vi "FolloWinDemo.vi"() -> ()   [LabVIEW 2023]
doc: "TOP VI of this project that demonstrates the use of \"FolloWin\" class. \n\nRun this VI to run the demo"
uses:
  FolloWin Class/FolloWin.lvclass
panel:
  in  "Intensity Graph":dbl[][](graph)
  in  "XY Graph":cluster{"X":dbl, "Y":dbl}[](graph)
  in  "Transparency":u8=30 max=100 step=1
  in  "Update\ndelay(ms)":u32=15 max=100000
  in  "Y offset":i32=30 min=-10000 max=10000
  in  "X offset":i32=30 min=-10000 max=10000
  in  "Width":u32=130 max=100000
  in  "Height":u32=50 max=100000
  # "FolloWin Demonstration VI"
  # "Description\n\nThis is a demonstration of the \"FolloWin\" Class. \nit's an object that implements an information window that follows the mouse cursor.\n\n\nTo use\n\nRun this VI and move the mouse  cursor over the \ngraphs.\n\nPress the mouse button to switch between position and line/measuring modes. \n\nTo stop the demonstration  use the X button on the top right."
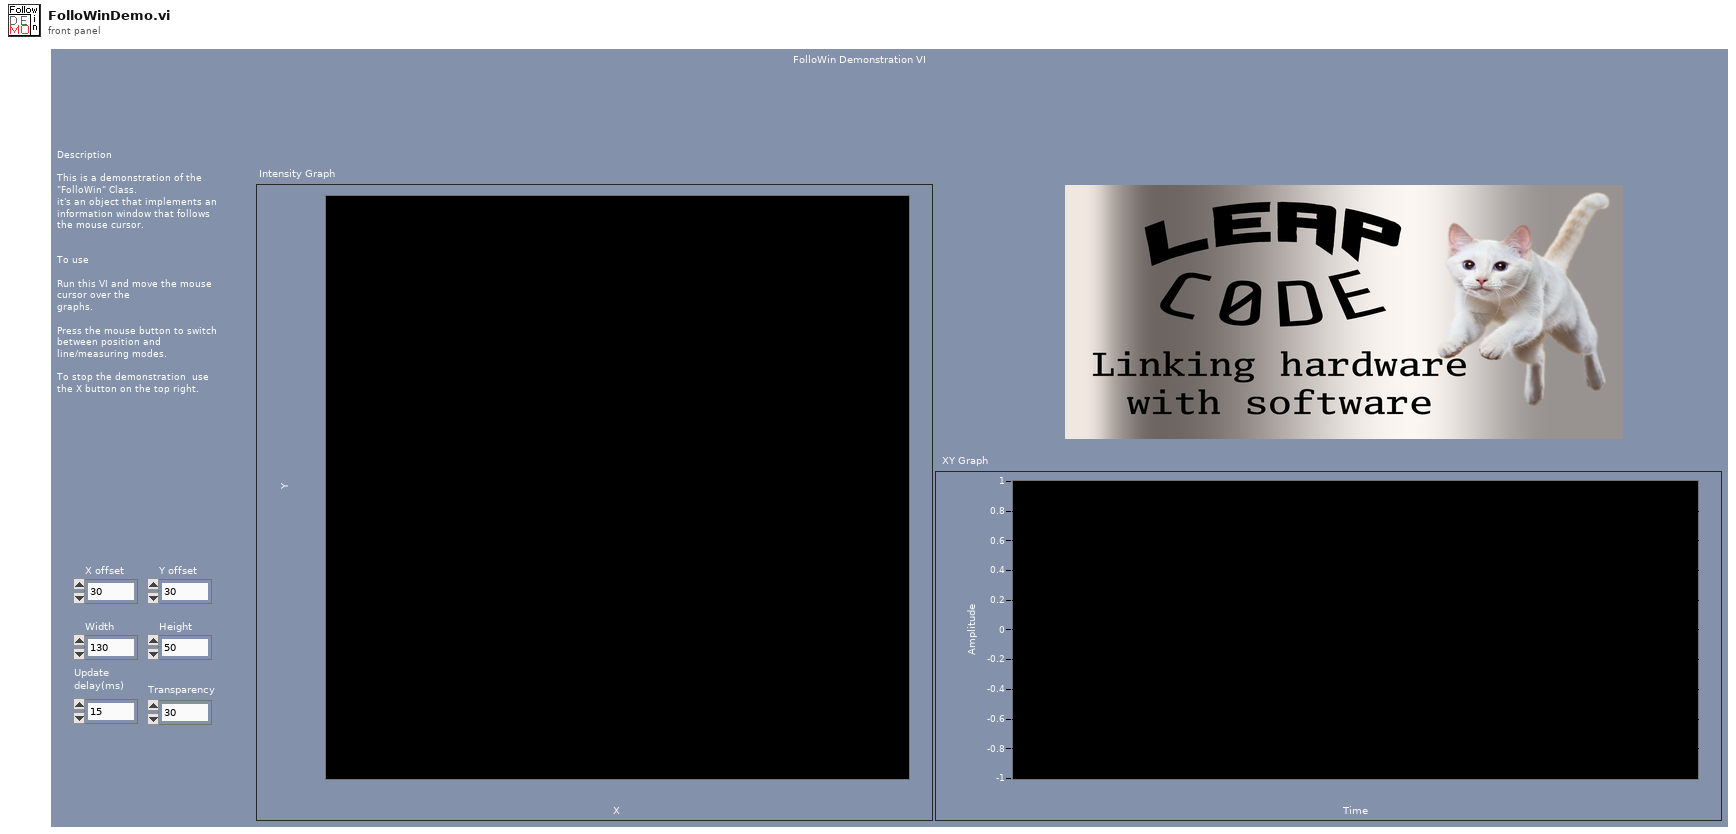
[diagram p1: front panel]
types:
  T1 = typedef "LVRectTypeDef.ctl" = cluster{"Left":i16, "Top":i16, "Right":i16, "Bottom":i16}
  T2 = typedef "LVPoint32TypeDef.ctl" = cluster{"Horizontal":i32, "Vertical":i32}
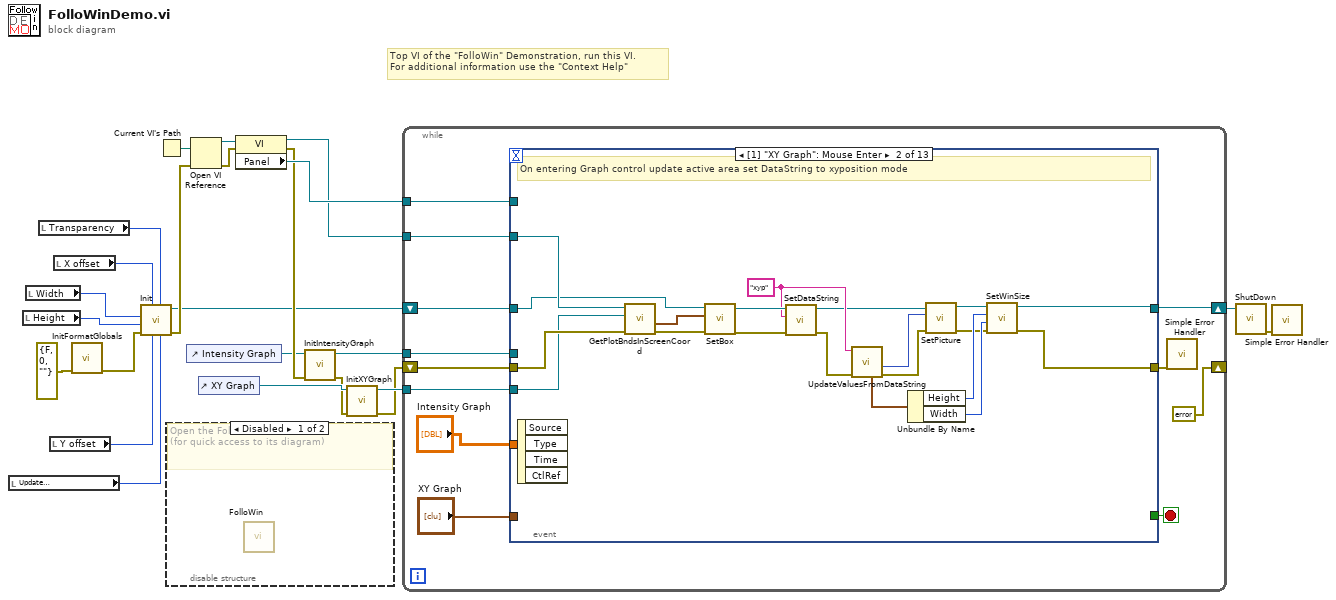
[diagram p0: block diagram]
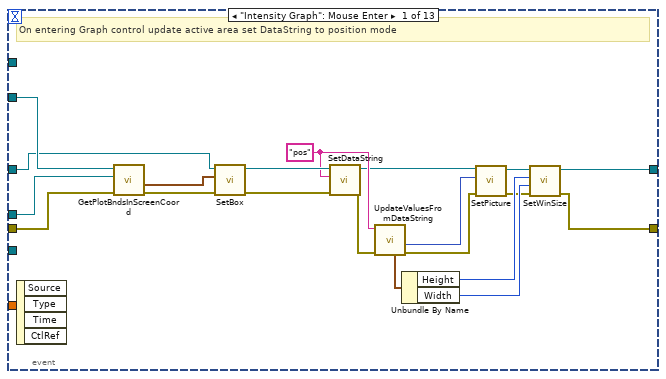
[diagram p3: hidden frame]
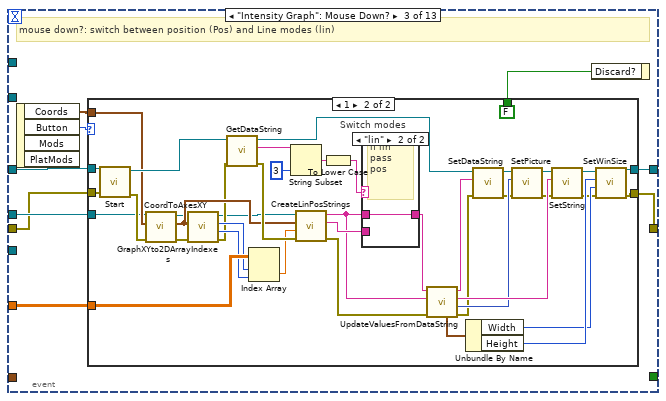
[diagram p4: hidden frame]
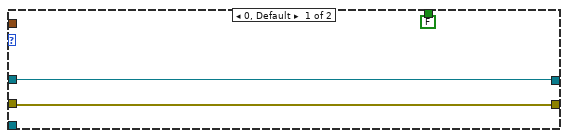
[diagram p5: hidden frame]
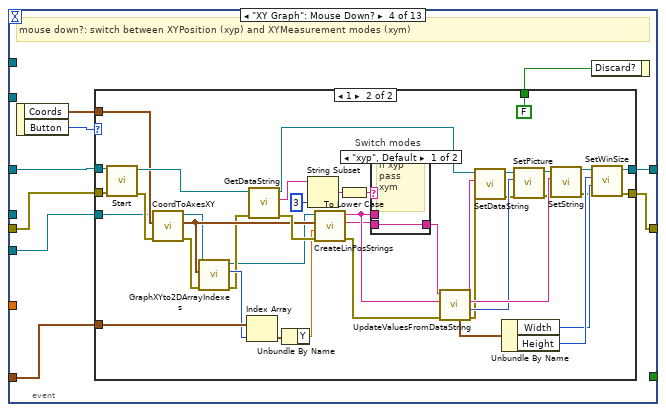
[diagram p7: hidden frame]
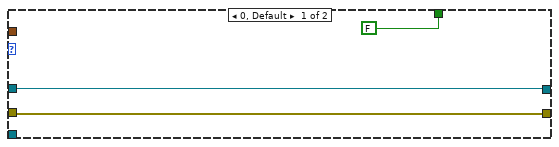
[diagram p8: hidden frame]
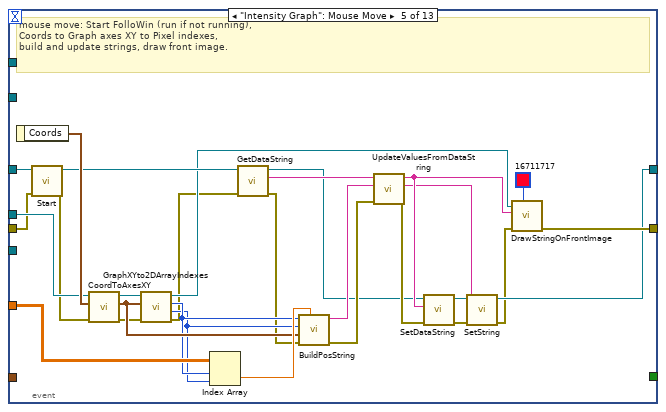
[diagram p10: hidden frame]
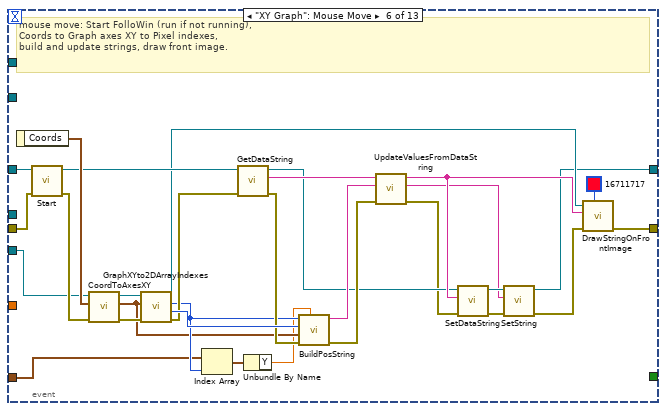
[diagram p11: hidden frame]
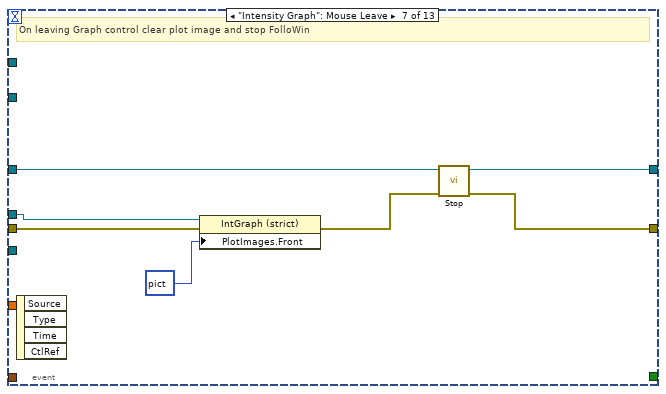
[diagram p12: hidden frame]
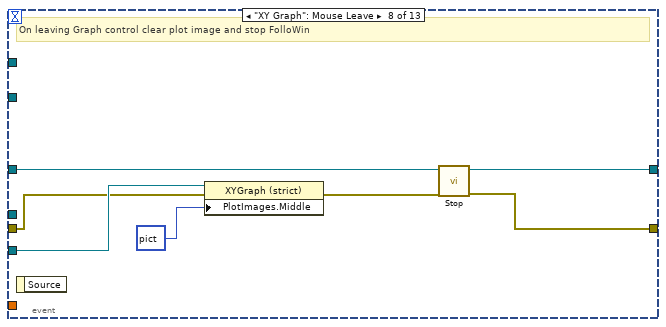
[diagram p13: hidden frame]
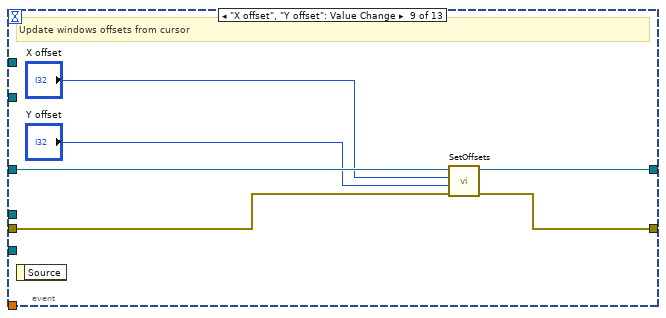
[diagram p14: hidden frame]
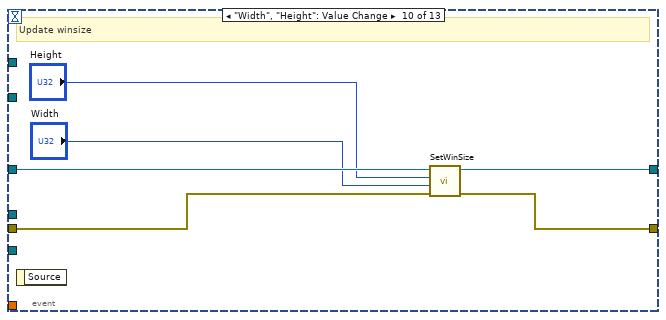
[diagram p15: hidden frame]
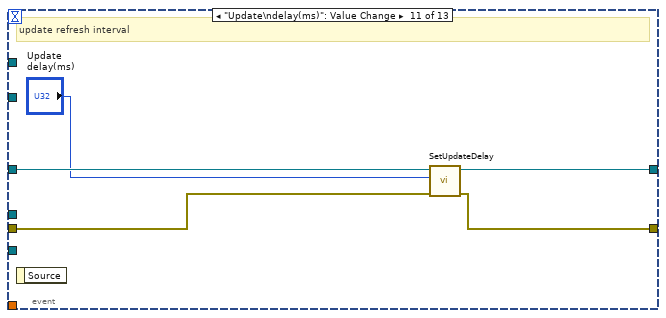
[diagram p16: hidden frame]
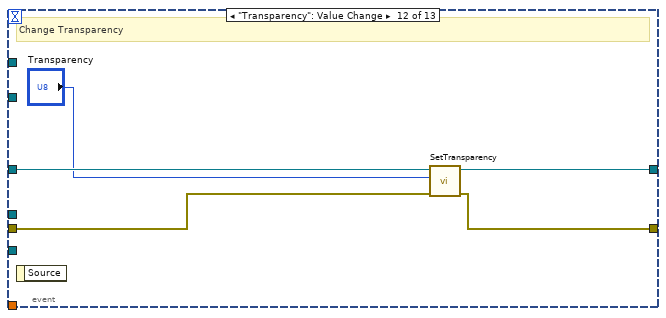
[diagram p17: hidden frame]
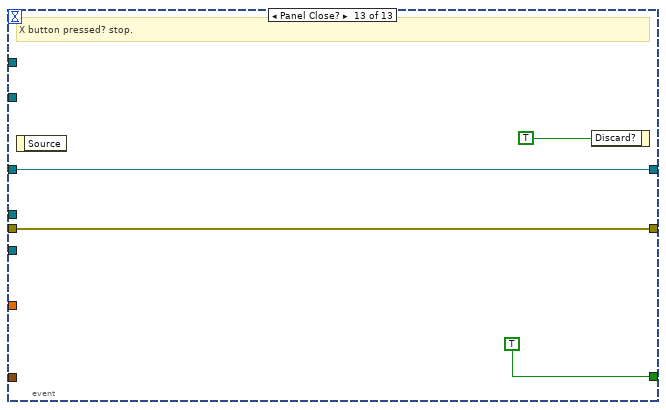
[diagram p18: hidden frame]
diagram:
  # "Top VI of the \"FolloWin\" Demonstration, run this VI. \nFor additional information use the \"Context Help\""
  n1 = local read "Update\ndelay(ms)"() -> (w12:u32)
  n2 = local read "Height"() -> (w23:u32)
  n3 = local read "Width"() -> (w24:u32)
  n4 = local read "Transparency"() -> (w11:u8)
  n5 = local read "Y offset"() -> (w17:i32)
  n6 = local read "X offset"() -> (w18:i32)
  n7 = call "InitFormatGlobals.vi"("error in (no error)"=errorcluster {"status"=FALSE, "code"=0, "source"=""}) -> ("error out"=w6:errorcluster)  [unwired: 10 in]
  n8 = call "Init.vi"("Update delay (ms)"=w12, "Transparency"=w11, "Y offset"=w17, "X offset"=w18, "error in (no error)"=w6, "WinHeight"=w23, "WinWidth"=w24) -> ("error out"=w15:errorcluster, "FolloWin out"=w10:refnum<class "FolloWin.lvclass">)  [unwired: 3 in]
  n9 = Current VI's Path() -> (path=w21:path)
  n10 = disable-structure "Diagram Disable Structure" shown="Disabled" {
    frame Disabled {
      # "Open the FolloWin GUI window\n(for quick access to its diagram)"
      n11 = call "FolloWin.vi"() -> ()  [unwired: 12 in]
    }
    frame Enabled {
    }
  }
  n12 = control-ref of="Intensity Graph"() -> (w1:refnum<vi>)
  n13 = Open VI Reference(vi path=w21, error in (no error)=w15) -> (vi reference=w20:refnum<vi>, error out=w16:errorcluster)  [unwired: 4 in]
  n14 = control-ref of="XY Graph"() -> (w5:refnum<vi>)
  n15 = property on="Property Node" class="VI"(reference=w20, error in=w16) -> (reference out=w13:refnum<vi>, error out=w14:errorcluster, "Panel"=w19:refnum<vi>)
  n16 = call "InitIntensityGraph.vi"("error in (no error)"=w14, "IntensityGraph in"=w1) -> ("error out"=w2:errorcluster, "IntensityGraph out"=w22:refnum<vi>)  [unwired: 8 in]
  n17 = call "InitXYGraph.vi"("error in (no error)"=w2, "XYGraph in"=w5) -> ("error out"=w3:errorcluster, "XYGraph out"=w4:refnum<vi>)  [unwired: 8 in]
  n18 = while {
    shift-right: [w35] -> w9
    shift-left: w10 -> [w36]
    shift-right: [errorcluster {"status"=FALSE, "code"=0, "source"=""} ("error out")] -> _
    shift-left: w3 -> [w34]
    tunnel: w22 -> [w32]
    tunnel: w19 -> [w31]
    tunnel: w13 -> [w30]
    tunnel: w4 -> [w27]
    stop <- w29 stop-if-true
    n19 = event shown="[1] \"XY Graph\": Mouse Enter" {
      selector: _ -> [_ _ _ _ _ _ _ _ _ _ _ _ _]
      dyn-events: _ -> [_ _ _ _ _ _ _ _ _ _ _ _ _]
      timeout: _ -> [_ _ _ _ _ _ _ _ _ _ _ _ _]
      tunnel: w36 -> [w52 w73 w85 w140 w211 w244 w250 w257 w265 w271 w276 w281 w282]
      tunnel: [w37 w66 w84 w139 w190 w218 w252 w259 w264 w266 w273 w278 w282] -> w35
      tunnel: w34 -> [w51 w72 w80 w137 w198 w233 w249 w255 w262 w268 w275 w280 w283]
      tunnel: [w46 w62 w77 w136 w191 w226 w251 w258 w263 w267 w274 w279 w283] -> w33
      tunnel: "Intensity Graph" -> [_ _ w81 _ w214 _ _ _ _ _ _ _ _]
      tunnel: w32 -> [w54 _ w82 _ w205 _ w247 _ _ _ _ _ _]
      tunnel: w31 -> [_ _ _ _ _ _ _ _ _ _ _ _ _]
      tunnel: w30 -> [w55 w75 _ _ _ _ _ _ _ _ _ _ _]
      tunnel: [_ _ _ _ _ _ _ _ _ _ _ _ TRUE] -> w29
      tunnel: w27 -> [_ w69 _ w133 _ w224 _ w256 _ _ _ _ _]
      tunnel: "XY Graph" -> [_ _ _ w132 _ w220 _ _ _ _ _ _ _]
      event "Intensity Graph": Mouse Enter {
        w48 = "pos" ("DataString")
        # "On entering Graph control update active area set DataString to position mode"
        n20 = event-data() -> ()  [unwired: 1 in, 4 out]
        n21 = call "GetPlotBndsInScreenCoord.vi"("error in (no error)"=w51, "IntensityGraph in"=w54, "VI in"=w55) -> ("error out"=w53:errorcluster, "Bounds Screen Coordinates"=w56:T1)  [unwired: 6 in, 1 out]
        n22 = call "SetBox.vi"("error in (no error)"=w53, "Box"=w56, "FolloWin in"=w52) -> ("error out"=w49:errorcluster, "FolloWin out"=w50:refnum<class "FolloWin.lvclass">)  [unwired: 7 in]
        n23 = call-dynamic "SetDataString.vi"("error in (no error)"=w49, "DataString"=w48, "FolloWin in"=w50) -> ("error out"=w47:errorcluster, "FolloWin out"=w41:refnum<class "FolloWin.lvclass">)  [unwired: 7 in]
        n24 = call "UpdateValuesFromDataString.vi"("error In"=w47, "Current String"=w48) -> ("error out"=w39:errorcluster, "BG Image"=w42:picture, "WinSize"=w45:cluster{"Width":i32, "Height":i32})  [unwired: 5 in, 2 out]
        n25 = Unbundle By Name(w45) -> ("Height"=w43:i32, "Width"=w44:i32)
        n26 = call-dynamic "SetPicture.vi"("error in (no error)"=w39, "Picture"=w42, "FolloWin in"=w41) -> ("error out"=w38:errorcluster, "FolloWin out"=w40:refnum<class "FolloWin.lvclass">)  [unwired: 7 in]
        n27 = call-dynamic "SetWinSize.vi"("error in (no error)"=w38, "Width"=w44, "Height"=w43, "FolloWin in"=w40) -> ("error out"=w46:errorcluster, "FolloWin out"=w37:refnum<class "FolloWin.lvclass">)  [unwired: 6 in]
      }
      event "XY Graph": Mouse Enter {
        w68 = "xyp" ("DataString")
        # "On entering Graph control update active area set DataString to xyposition mode"
        n28 = event-data() -> ()  [unwired: 1 in, 4 out]
        n29 = call "GetPlotBndsInScreenCoord.vi"("error in (no error)"=w72, "IntensityGraph in"=w69, "VI in"=w75) -> ("error out"=w74:errorcluster, "Bounds Screen Coordinates"=w76:T1)  [unwired: 6 in, 1 out]
        n30 = call "SetBox.vi"("error in (no error)"=w74, "Box"=w76, "FolloWin in"=w73) -> ("error out"=w70:errorcluster, "FolloWin out"=w71:refnum<class "FolloWin.lvclass">)  [unwired: 7 in]
        n31 = call-dynamic "SetDataString.vi"("error in (no error)"=w70, "DataString"=w68, "FolloWin in"=w71) -> ("error out"=w67:errorcluster, "FolloWin out"=w61:refnum<class "FolloWin.lvclass">)  [unwired: 7 in]
        n32 = call "UpdateValuesFromDataString.vi"("error In"=w67, "Current String"=w68) -> ("error out"=w58:errorcluster, "BG Image"=w59:picture, "WinSize"=w65:cluster{"Width":i32, "Height":i32})  [unwired: 5 in, 2 out]
        n33 = Unbundle By Name(w65) -> ("Height"=w63:i32, "Width"=w64:i32)
        n34 = call-dynamic "SetPicture.vi"("error in (no error)"=w58, "Picture"=w59, "FolloWin in"=w61) -> ("error out"=w57:errorcluster, "FolloWin out"=w60:refnum<class "FolloWin.lvclass">)  [unwired: 7 in]
        n35 = call-dynamic "SetWinSize.vi"("error in (no error)"=w57, "Width"=w64, "Height"=w63, "FolloWin in"=w60) -> ("error out"=w62:errorcluster, "FolloWin out"=w66:refnum<class "FolloWin.lvclass">)  [unwired: 6 in]
      }
      event "Intensity Graph": Mouse Down? {
        # "mouse down?: switch between position (Pos) and Line modes (lin)"
        n36 = event-data() -> ("Coords"=w83:T2, "Button"=w79:u16)  [unwired: 1 in, 2 out]
        n37 = case shown="1" w79 {
          tunnel: w85 -> [w88 w127]
          tunnel: [w88 w92] -> w84
          tunnel: w83 -> [_ w125]
          tunnel: w82 -> [_ w110]
          tunnel: w81 -> [_ w115]
          tunnel: w80 -> [w86 w119]
          tunnel: [FALSE ("Discard?") FALSE ("Discard?")] -> w78
          tunnel: [w86 w93] -> w77
          frame 0, Default {
          }
          frame 1 {
            n38 = call "Start.vi"("error in (no error)"=w119, "FolloWin in"=w127) -> ("error out"=w118:errorcluster, "FolloWin out"=w129:refnum<class "FolloWin.lvclass">)  [unwired: 8 in]
            n39 = call "CoordToAxesXY.vi"("error in (no error)"=w118, "Coords"=w125, "IntensityGraph in"=w110) -> ("error out"=w109:errorcluster, "XY"=w113:cluster{"X":dbl, "Y":dbl}, "IntensityGraph out"=w107:refnum<vi>)  [unwired: 6 in]
            n40 = call "GraphXYto2DArrayIndexes.vi"("error in (no error)"=w109, "XY"=w113, "IntensityGraph in"=w107) -> ("error out"=w108:errorcluster, "Y Index"=w111:i32, "X Index"=w112:i32, "reference out"=w106:refnum<vi>)  [unwired: 5 in]
            n41 = call-dynamic "GetDataString.vi"("error in (no error)"=w108, "FolloWin in"=w129) -> ("error out"=w126:errorcluster, "DataString"=w123:string, "FolloWin out"=w97:refnum<class "FolloWin.lvclass">)  [unwired: 7 in]
            n42 = Index Array(array=w115, index (row)=w112, index (col)=w111) -> (element=w114:dbl)
            n43 = String Subset(string=w123, length (rest)=3 ("length (rest)")) -> (substring=w104:string)  [unwired: 1 in]
            n44 = call "CreateLinPosStrings.vi"("error in (no error)"=w126, "Z/F(x) val"=w114, "Coord"=w113, "IntensityGraph in"=w106) -> ("error out"=w117:errorcluster, "Lin String out"=w121:string, "Pos String out"=w105:string)  [unwired: 5 in]
            n45 = To Lower Case(string=w104) -> (all lower case string=w103:string)
            n46 = case "Switch modes" shown="\"lin\"" w103 {
              tunnel: w121 -> [w130 _]
              tunnel: [w130 w131] -> w120
              tunnel: w105 -> [_ w131]
              frame "pos", Default {
                # "if pos\npass lin"
              }
              frame "lin" {
                # "if lin \npass pos"
              }
            }
            n47 = call "UpdateValuesFromDataString.vi"("error In"=w117, "New point string"=w105, "Current String"=w120) -> ("error out"=w95:errorcluster, "BG Image"=w101:picture, "DisplayString"=w124:string, "DataString"=w128:string, "WinSize"=w100:cluster{"Width":i32, "Height":i32})  [unwired: 4 in]
            n48 = Unbundle By Name(w100) -> ("Width"=w98:i32, "Height"=w99:i32)
            n49 = call-dynamic "SetDataString.vi"("error in (no error)"=w95, "DataString"=w128, "FolloWin in"=w97) -> ("error out"=w96:errorcluster, "FolloWin out"=w89:refnum<class "FolloWin.lvclass">)  [unwired: 7 in]
            n50 = call-dynamic "SetPicture.vi"("error in (no error)"=w96, "Picture"=w101, "FolloWin in"=w89) -> ("error out"=w102:errorcluster, "FolloWin out"=w90:refnum<class "FolloWin.lvclass">)  [unwired: 7 in]
            n51 = call-dynamic "SetString.vi"("error in (no error)"=w102, "String Text"=w124, "FolloWin in"=w90) -> ("error out"=w94:errorcluster, "FolloWin out"=w91:refnum<class "FolloWin.lvclass">)  [unwired: 7 in]
            n52 = call-dynamic "SetWinSize.vi"("error in (no error)"=w94, "Width"=w98, "Height"=w99, "FolloWin in"=w91) -> ("error out"=w93:errorcluster, "FolloWin out"=w92:refnum<class "FolloWin.lvclass">)  [unwired: 6 in]
          }
        }
        n53 = event-data ("Event Filter Node")("Discard?"=w78) -> ()  [unwired: 1 in, 1 out]
      }
      event "XY Graph": Mouse Down? {
        # "mouse down?: switch between XYPosition (xyp) and XYMeasurement modes (xym)"
        n54 = event-data() -> ("Coords"=w138:T2, "Button"=w135:u16)  [unwired: 1 in]
        n55 = case shown="1" w135 {
          tunnel: w140 -> [w143 w182]
          tunnel: [w143 w154] -> w139
          tunnel: w138 -> [_ w180]
          tunnel: w133 -> [_ w168]
          tunnel: w137 -> [w142 w176]
          tunnel: [w142 w155] -> w136
          tunnel: [FALSE ("Discard?") FALSE ("Discard?")] -> w134
          tunnel: w132 -> [_ w172]
          frame 0, Default {
          }
          frame 1 {
            n56 = call "Start.vi"("error in (no error)"=w176, "FolloWin in"=w182) -> ("error out"=w175:errorcluster, "FolloWin out"=w184:refnum<class "FolloWin.lvclass">)  [unwired: 8 in]
            n57 = call "CoordToAxesXY.vi"("error in (no error)"=w175, "Coords"=w180, "IntensityGraph in"=w168) -> ("error out"=w166:errorcluster, "XY"=w169:cluster{"X":dbl, "Y":dbl}, "IntensityGraph out"=w164:refnum<vi>)  [unwired: 6 in]
            n58 = call "GraphXYto2DArrayIndexes.vi"("error in (no error)"=w166, "XY"=w169, "IntensityGraph in"=w164) -> ("error out"=w165:errorcluster, "X Index"=w167:i32, "reference out"=w163:refnum<vi>)  [unwired: 5 in, 1 out]
            n59 = Index Array(array=w172, index=w167) -> (element=w171:cluster{"X":dbl, "Y":dbl})
            n60 = call-dynamic "GetDataString.vi"("error in (no error)"=w165, "FolloWin in"=w184) -> ("error out"=w181:errorcluster, "DataString"=w178:string, "FolloWin out"=w149:refnum<class "FolloWin.lvclass">)  [unwired: 7 in]
            n61 = Unbundle By Name(w171) -> ("Y"=w170:dbl)
            n62 = String Subset(string=w178, length (rest)=3 ("length (rest)")) -> (substring=w162:string)  [unwired: 1 in]
            n63 = call "CreateLinPosStrings.vi"("error in (no error)"=w181, "Z/F(x) val"=w170, "Coord"=w169, "IntensityGraph in"=w163) -> ("error out"=w174:errorcluster, "Lin String out"=w145:string, "Pos String out"=w146:string)  [unwired: 5 in]
            n64 = To Lower Case(string=w162) -> (all lower case string=w147:string)
            n65 = case "Switch modes" shown="\"xyp\", Default" w147 {
              tunnel: w145 -> [w185 _]
              tunnel: [w185 w186] -> w144
              tunnel: w146 -> [_ w186]
              frame "xyp", Default {
                # "if xyp pass xym"
              }
              frame "xym" {
                # "if xym \npass xyp"
              }
            }
            n66 = call "UpdateValuesFromDataString.vi"("error In"=w174, "New point string"=w146, "Current String"=w144) -> ("error out"=w148:errorcluster, "BG Image"=w160:picture, "DisplayString"=w179:string, "DataString"=w183:string, "WinSize"=w156:cluster{"Width":i32, "Height":i32})  [unwired: 4 in]
            n67 = call-dynamic "SetDataString.vi"("error in (no error)"=w148, "DataString"=w183, "FolloWin in"=w149) -> ("error out"=w151:errorcluster, "FolloWin out"=w150:refnum<class "FolloWin.lvclass">)  [unwired: 7 in]
            n68 = Unbundle By Name(w156) -> ("Width"=w157:i32, "Height"=w158:i32)
            n69 = call-dynamic "SetPicture.vi"("error in (no error)"=w151, "Picture"=w160, "FolloWin in"=w150) -> ("error out"=w159:errorcluster, "FolloWin out"=w161:refnum<class "FolloWin.lvclass">)  [unwired: 7 in]
            n70 = call-dynamic "SetString.vi"("error in (no error)"=w159, "String Text"=w179, "FolloWin in"=w161) -> ("error out"=w152:errorcluster, "FolloWin out"=w153:refnum<class "FolloWin.lvclass">)  [unwired: 7 in]
            n71 = call-dynamic "SetWinSize.vi"("error in (no error)"=w152, "Width"=w157, "Height"=w158, "FolloWin in"=w153) -> ("error out"=w155:errorcluster, "FolloWin out"=w154:refnum<class "FolloWin.lvclass">)  [unwired: 6 in]
          }
        }
        n72 = event-data ("Event Filter Node")("Discard?"=w134) -> ()  [unwired: 1 in, 1 out]
      }
      event "Intensity Graph": Mouse Move {
        # "mouse move: Start FolloWin (run if not running), \nCoords to Graph axes XY to Pixel indexes, \nbuild and update strings, draw front image."
        n73 = event-data() -> ("Coords"=w215:T2)  [unwired: 1 in]
        n74 = call "Start.vi"("error in (no error)"=w198, "FolloWin in"=w211) -> ("error out"=w197:errorcluster, "FolloWin out"=w207:refnum<class "FolloWin.lvclass">)  [unwired: 8 in]
        n75 = call "CoordToAxesXY.vi"("error in (no error)"=w197, "Coords"=w215, "IntensityGraph in"=w205) -> ("error out"=w199:errorcluster, "XY"=w212:cluster{"X":dbl, "Y":dbl}, "IntensityGraph out"=w203:refnum<vi>)  [unwired: 6 in]
        n76 = call "GraphXYto2DArrayIndexes.vi"("error in (no error)"=w199, "XY"=w212, "IntensityGraph in"=w203) -> ("error out"=w196:errorcluster, "Y Index"=w209:i32, "X Index"=w210:i32, "reference out"=w202:refnum<vi>)  [unwired: 5 in]
        n77 = Index Array(array=w214, index (row)=w210, index (col)=w209) -> (element=w213:dbl)
        n78 = call-dynamic "GetDataString.vi"("error in (no error)"=w196, "FolloWin in"=w207) -> ("error out"=w195:errorcluster, "DataString"=w206:string, "FolloWin out"=w187:refnum<class "FolloWin.lvclass">)  [unwired: 7 in]
        n79 = call "BuildPosString.vi"("Z val"=w213, "error in (no error)"=w195, "XY"=w212, "Y graph pixels"=w209, "X graph pixels"=w210) -> ("error out"=w194:errorcluster, "String"=w208:string)  [unwired: 5 in]
        n80 = call "UpdateValuesFromDataString.vi"("error In"=w194, "New point string"=w208, "Current String"=w206) -> ("error out"=w188:errorcluster, "DisplayString"=w200:string, "DataString"=w204:string)  [unwired: 4 in, 2 out]
        n81 = call-dynamic "SetDataString.vi"("error in (no error)"=w188, "DataString"=w204, "FolloWin in"=w187) -> ("error out"=w192:errorcluster, "FolloWin out"=w201:refnum<class "FolloWin.lvclass">)  [unwired: 7 in]
        n82 = call-dynamic "SetString.vi"("error in (no error)"=w192, "String Text"=w200, "FolloWin in"=w201) -> ("error out"=w189:errorcluster, "FolloWin out"=w190:refnum<class "FolloWin.lvclass">)  [unwired: 7 in]
        n83 = call "DrawStringOnFrontImage.vi"("color(black)"=u32 16711717, "error in"=w189, "input string"=w204, "Graph Ref"=w202) -> ("error out"=w191:errorcluster)  [unwired: 6 in, 1 out]
      }
      event "XY Graph": Mouse Move {
        # "mouse move: Start FolloWin (run if not running), \nCoords to Graph axes XY to Pixel indexes, \nbuild and update strings, draw front image."
        n84 = event-data() -> ("Coords"=w245:T2)  [unwired: 1 in]
        n85 = call "Start.vi"("error in (no error)"=w233, "FolloWin in"=w244) -> ("error out"=w232:errorcluster, "FolloWin out"=w241:refnum<class "FolloWin.lvclass">)  [unwired: 8 in]
        n86 = call "CoordToAxesXY.vi"("error in (no error)"=w232, "Coords"=w245, "IntensityGraph in"=w224) -> ("error out"=w234:errorcluster, "XY"=w223:cluster{"X":dbl, "Y":dbl}, "IntensityGraph out"=w238:refnum<vi>)  [unwired: 6 in]
        n87 = call "GraphXYto2DArrayIndexes.vi"("error in (no error)"=w234, "XY"=w223, "IntensityGraph in"=w238) -> ("error out"=w231:errorcluster, "Y Index"=w243:i32, "X Index"=w225:i32, "reference out"=w237:refnum<vi>)  [unwired: 5 in]
        n88 = Index Array(array=w220, index=w225) -> (element=w222:cluster{"X":dbl, "Y":dbl})
        n89 = call-dynamic "GetDataString.vi"("error in (no error)"=w231, "FolloWin in"=w241) -> ("error out"=w230:errorcluster, "DataString"=w240:string, "FolloWin out"=w217:refnum<class "FolloWin.lvclass">)  [unwired: 7 in]
        n90 = Unbundle By Name(w222) -> ("Y"=w221:dbl)
        n91 = call "BuildPosString.vi"("Z val"=w221, "error in (no error)"=w230, "XY"=w223, "Y graph pixels"=w243, "X graph pixels"=w225) -> ("error out"=w229:errorcluster, "String"=w242:string)  [unwired: 5 in]
        n92 = call "UpdateValuesFromDataString.vi"("error In"=w229, "New point string"=w242, "Current String"=w240) -> ("error out"=w216:errorcluster, "DisplayString"=w235:string, "DataString"=w239:string)  [unwired: 4 in, 2 out]
        n93 = call-dynamic "SetDataString.vi"("error in (no error)"=w216, "DataString"=w239, "FolloWin in"=w217) -> ("error out"=w227:errorcluster, "FolloWin out"=w236:refnum<class "FolloWin.lvclass">)  [unwired: 7 in]
        n94 = call-dynamic "SetString.vi"("error in (no error)"=w227, "String Text"=w235, "FolloWin in"=w236) -> ("error out"=w219:errorcluster, "FolloWin out"=w218:refnum<class "FolloWin.lvclass">)  [unwired: 7 in]
        n95 = call "DrawStringOnFrontImage.vi"("color(black)"=u32 16711717, "error in"=w219, "input string"=w239, "Graph Ref"=w237) -> ("error out"=w226:errorcluster)  [unwired: 6 in, 1 out]
      }
      event "Intensity Graph": Mouse Leave {
        # "On leaving Graph control clear plot image and stop FolloWin"
        n96 = event-data() -> ()  [unwired: 1 in, 4 out]
        n97 = property class="IntGraph (strict)"(reference=w247, error in=w249, "PlotImages.Front"=picture data[5B] ("Plot Images:Front")) -> (error out=w248:errorcluster)  [unwired: 1 out]
        n98 = call-dynamic "Stop.vi"("error in (no error)"=w248, "FolloWin in"=w250) -> ("error out"=w251:errorcluster, "FolloWin out"=w252:refnum<class "FolloWin.lvclass">)  [unwired: 8 in]
      }
      event "XY Graph": Mouse Leave {
        # "On leaving Graph control clear plot image and stop FolloWin"
        n99 = event-data() -> ()  [unwired: 1 in, 1 out]
        n100 = property class="XYGraph (strict)"(reference=w256, error in=w255, "PlotImages.Middle"=picture data[5B] ("Plot Images:Front")) -> (error out=w254:errorcluster)  [unwired: 1 out]
        n101 = call-dynamic "Stop.vi"("error in (no error)"=w254, "FolloWin in"=w257) -> ("error out"=w258:errorcluster, "FolloWin out"=w259:refnum<class "FolloWin.lvclass">)  [unwired: 8 in]
      }
      event "X offset", "Y offset": Value Change {
        # "Update windows offsets from cursor"
        n102 = event-data() -> ()  [unwired: 1 in, 1 out]
        n103 = call-dynamic "SetOffsets.vi"("error in (no error)"=w262, "Y offset"="Y offset", "X offset"="X offset", "FolloWin in"=w265) -> ("error out"=w263:errorcluster, "FolloWin out"=w264:refnum<class "FolloWin.lvclass">)  [unwired: 6 in]
      }
      event "Width", "Height": Value Change {
        # "Update winsize"
        n104 = event-data() -> ()  [unwired: 1 in, 1 out]
        n105 = call-dynamic "SetWinSize.vi"("error in (no error)"=w268, "Width"="Width", "Height"="Height", "FolloWin in"=w271) -> ("error out"=w267:errorcluster, "FolloWin out"=w266:refnum<class "FolloWin.lvclass">)  [unwired: 6 in]
      }
      event "Update\ndelay(ms)": Value Change {
        # "update refresh interval"
        n106 = event-data() -> ()  [unwired: 1 in, 1 out]
        n107 = call-dynamic "SetUpdateDelay.vi"("error in (no error)"=w275, "Update delay (ms)"="Update\ndelay(ms)", "FolloWin in"=w276) -> ("error out"=w274:errorcluster, "FolloWin out"=w273:refnum<class "FolloWin.lvclass">)  [unwired: 7 in]
      }
      event "Transparency": Value Change {
        # "Change Transparency"
        n108 = event-data() -> ()  [unwired: 1 in, 1 out]
        n109 = call-dynamic "SetTransparency.vi"("error in (no error)"=w280, "Transparency"="Transparency", "FolloWin in"=w281) -> ("error out"=w279:errorcluster, "FolloWin out"=w278:refnum<class "FolloWin.lvclass">)  [unwired: 7 in]
      }
      event Panel Close? {
        # "X button pressed? stop."
        n110 = event-data() -> ()  [unwired: 1 in, 1 out]
        n111 = event-data ("Event Filter Node")("Discard?"=TRUE) -> ()  [unwired: 1 in, 1 out]
      }
    }
    n112 = call <vilib>:"Simple Error Handler.vi"("error in (no error)"=w33) -> ()  [unwired: 4 in, 5 out]
  }
  n113 = call-dynamic "ShutDown.vi"("FolloWin in"=w9) -> ("error out"=w8:errorcluster)  [unwired: 10 in]
  n114 = call <vilib>:"Simple Error Handler.vi"("error in (no error)"=w8) -> ()  [unwired: 4 in, 5 out]
